vi "Load Settings from XML.vi"(8 "error in":errorcluster, 11 "Settings in":T1) -> (0 "error out":errorcluster, 2 "all rows":string[][](array[string]), 3 "Settings out":T1)   [LabVIEW 2026, in "Settings.lvlib"]
doc: "Attempts to load previous user specified settings from an XML file.\n\nThis VI will not generate an error. If a suitable XML file can't be loaded and parsed then it will simply return the default settings."
uses:
  Settings.lvlib
  Settings.ctl
  Acquisition/Hardware Configuration.ctl
  Logging/Logging Configuration.ctl
  Acquisition/Acquisition.lvlib
  Logging/Logging.lvlib
panel:
  # "(Scroll up for Settings Controls)"
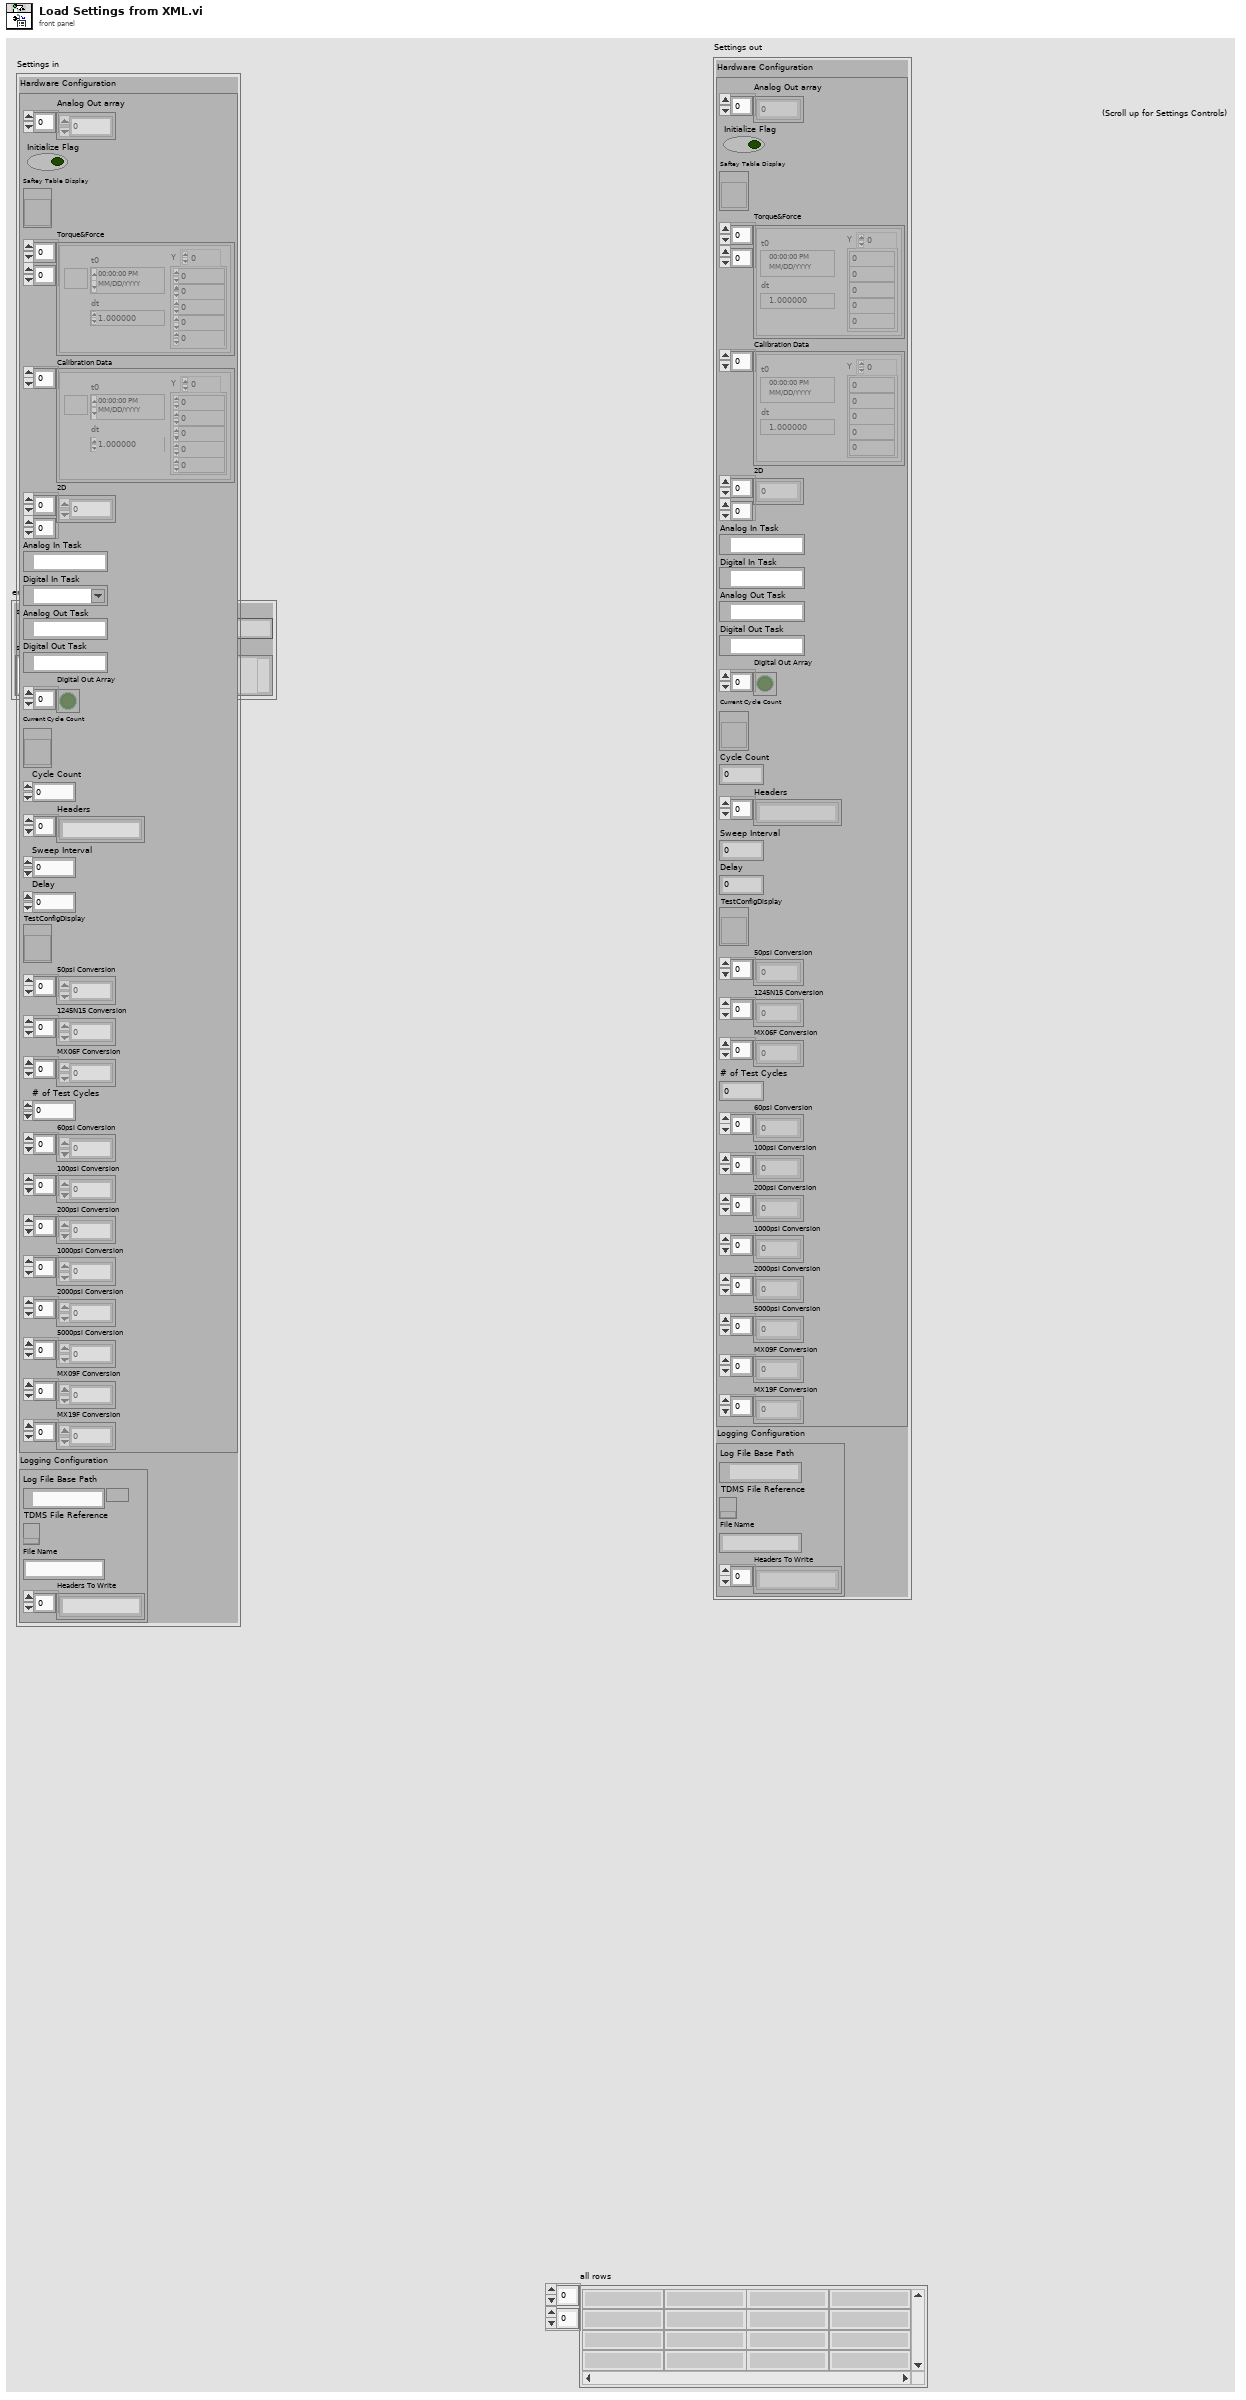
[diagram p1: front panel]
types:
  T1 = typedef "Settings.lvlib/Settings.ctl" = cluster{"Hardware Configuration":T2, "Logging Configuration":T3}
  T2 = typedef "Acquisition.lvlib/Hardware Configuration.ctl" = cluster{"Analog Out array":dbl[], "Initialize Flag":bool, "Saftey Table Display":refnum<vi>, "Torque&Force":waveform(dbl)[][], "Calibration Data":waveform(dbl)[], "2D":dbl[][], "Analog In Task":refnum<k21>, "Digital In Task":refnum<k21>, "Analog Out Task":refnum<k21>, "Digital Out Task":refnum<k21>, "Digital Out Array":bool[], "Current Cycle Count":refnum<vi>, "Cycle Count":u64, "Headers":string[], "Sweep Interval":u64, "Delay":u64, "TestConfigDisplay":refnum<vi>, "50psi Conversion":dbl[], "1245N15 Conversion":dbl[], "MX06F Conversion":dbl[], "# of Test Cycles":u64, "60psi Conversion":dbl[], "100psi Conversion":dbl[], "200psi Conversion":dbl[], "1000psi Conversion":dbl[], "2000psi Conversion":dbl[], "5000psi Conversion":dbl[], "MX09F Conversion":dbl[], "MX19F Conversion":dbl[]}
  T3 = typedef "Logging.lvlib/Logging Configuration.ctl" = cluster{"Log File Base Path":path, "TDMS File Reference":refnum<k34>, "File Name":string, "Headers To Write":string[]}
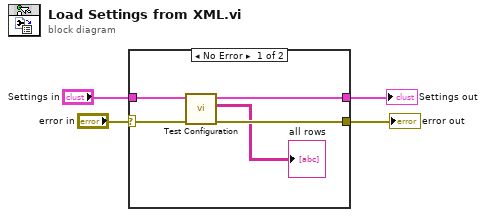
[diagram p0: block diagram]
diagram:
  n1 = case shown="No Error" "error in" {
    selector: "error in" -> [w9 w11]
    tunnel: [w8 w11] -> w3
    tunnel: "Settings in" -> [w6 w10]
    tunnel: [w5 w10] -> w1
    frame No Error {
      n2 = call "Test Configuration.vi"("error in (no error)"=w9, "Settings in"=w6) -> ("error out"=w8:errorcluster, "all rows"=→"all rows":string[][], "output cluster"=w5:T1)  [unwired: 7 in]
    }
    frame Error {
    }
  }
  "error out" <- w3
  "Settings out" <- w1
